vi "FiberSpectrograph_logEvent_simulationMode.vi"(8 "error in (no error)":errorcluster, 11 "logevent_simulationMode_Ctl":T1) -> (0 "error out":errorcluster, 2 "function return":i32, 3 "logevent_simulationMode_Ctl out":T1)   [LabVIEW 2016, in "SALLV_FiberSpectrograph.lvlib"]
doc: "int FiberSpectrograph_shm_logEvent_simulationModeLV(FiberSpectrograph_logevent_simulationModeLV *logevent_simulationMode_Ctl );"
uses:
  SALLV_FiberSpectrograph.lvlib
  DataTypes/logevent_simulationMode.ctl
  SALLV_FiberSpectrograph.so
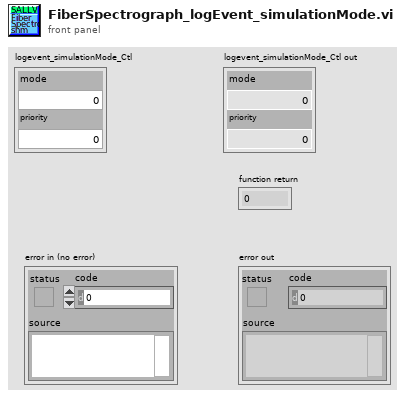
[diagram p1: front panel]
types:
  T1 = typedef "SALLV_FiberSpectrograph.lvlib/logevent_simulationMode.ctl" = cluster{"mode":i32, "priority":i32}
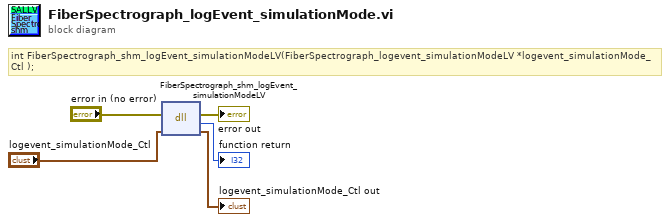
[diagram p0: block diagram]
diagram:
  # "int FiberSpectrograph_shm_logEvent_simulationModeLV(FiberSpectrograph_logevent_simulationModeLV *logevent_simulationMode_Ctl );"
  n1 = dll-call lib="home/harini/SALLV_FiberSpectrograph/SALLV_FiberSpectrograph.*" fn="FiberSpectrograph_shm_logEvent_simulationModeLV"(error in="error in (no error)", "logevent_simulationMode_Ctl"="logevent_simulationMode_Ctl") -> (error out=→"error out":errorcluster, →"function return":i32, "logevent_simulationMode_Ctl"=→"logevent_simulationMode_Ctl out":T1)  [unwired: 2 in, 1 out]
